vi "Get Next Node.vi"(8 "error in (no error)":errorcluster, 9 "State":string, 10 "Direction":enum16{"L", "R"}(ring), 11 "Network in":refnum<class "Stateless Network.lvclass">) -> (0 "error out":errorcluster, 2 "Node":string, 3 "Network out":refnum<class "Stateless Network.lvclass">)   [LabVIEW 2020, in "Stateless Network.lvclass"]
uses:
  Stateless Network.lvclass
  Stateless Network.lvclass/Stateless Network.ctl
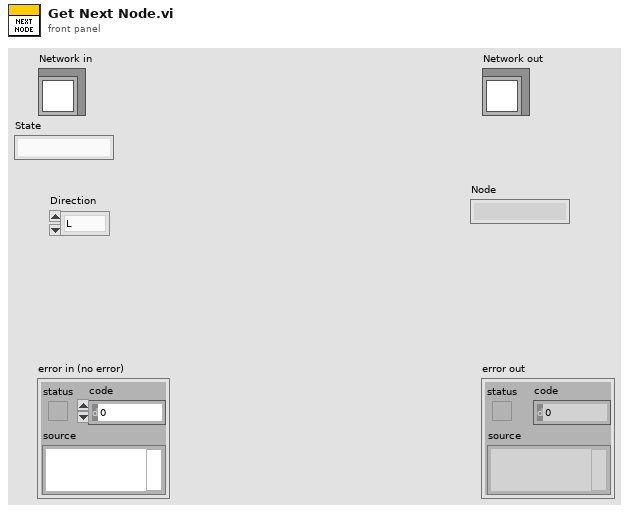
[diagram p1: front panel]
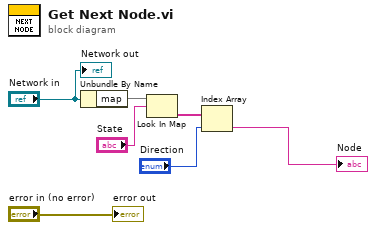
[diagram p0: block diagram]
diagram:
  n1 = Unbundle By Name("Network in") -> ("map"=w5:map{string, string[]})
  n2 = Look In Map(map=w5, key="State") -> (value=w4:string[])  [unwired: 1 in, 1 out]
  n3 = Index Array(array=w4, index="Direction") -> (element=→"Node":string)
  "error out" <- "error in (no error)"
  "Network out" <- "Network in"
